vi "启动整机测试 (子VI).vi"() -> (0 "error out":T1={"status"=FALSE, "代码"=4, "source"=""} caption="错误输出" {"代码" items=["执行成功"=1, "执行失败，但不知道原因"=2, "命令请求条件错误"=3, "通讯超时"=4, "系统繁忙不能执行"=5, "系统故障"=6, "没有数据"=100]})   [LabVIEW 2016, in "MB SLAVE.lvlib"]
uses:
  MB SLAVE.lvlib
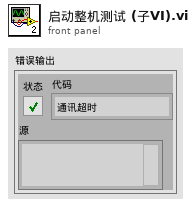
[diagram p1: front panel]
types:
  T1 = cluster{"status":bool, "代码":u16, "source":string}
  T2 = typedef "系统交互.ctl" = cluster{"运行模式":enum16{"维护模式", "常规模式", "应急模式", "质控模式"}, "运行间隔":i16, "流程运行中":bool, "自动运行启动参数":bool[], "SYSTEM Interface.总磷总氮类型":enum16{"单模块", "总磷总氮二合一模块", "氨氮总磷二合一模块"}, "多参数运行间隔":i16}
  T3 = cluster{"参数启用":cluster{"氨氮":bool, "总磷":bool, "总氮":bool, "多参数":bool, "CODMn":bool, "CODcr":bool, "超标留样":bool}}
  T4 = cluster{"自动运行启动参数[0]":bool, "自动运行启动参数[1]":bool, "自动运行启动参数[2]":bool, "自动运行启动参数[3]":bool, "自动运行启动参数[4]":bool, "自动运行启动参数[5]":bool, "自动运行启动参数[6]":bool}
  T5 = cluster{"自动运行启动参数":cluster{"自动运行启动参数[0]":bool, "自动运行启动参数[1]":bool, "自动运行启动参数[2]":bool, "自动运行启动参数[3]":bool, "自动运行启动参数[4]":bool, "自动运行启动参数[5]":bool, "自动运行启动参数[6]":bool}}
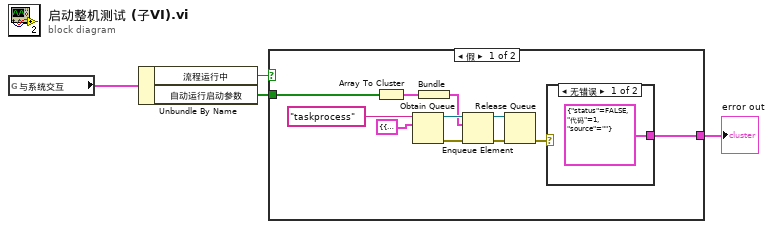
[diagram p0: block diagram]
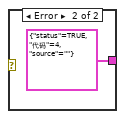
[diagram p2: hidden frame]
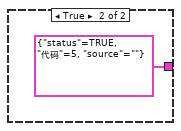
[diagram p3: hidden frame]
diagram:
  n1 = global read "modbus slave全局.vi" "与系统交互"() -> (w3:T2)
  n2 = Unbundle By Name(w3) -> ("流程运行中"=w2:bool, "自动运行启动参数"=w1:bool[])
  n3 = case shown="假" w2 {
    tunnel: [w15 T1 {"status"=TRUE, "代码"=5, "source"=""} ("error out")] -> w4
    tunnel: w1 -> [w6 _]
    frame False {
      n4 = Array To Cluster(array=w6) -> (cluster=w5:T4)
      n5 = Obtain Queue(name (unnamed)="taskprocess" ("名称（未命名）"), element data type=T3 {"参数启用"={"氨氮"=FALSE, "总磷"=FALSE, "总氮"=FALSE, "多参数"=FALSE, "CODMn"=FALSE, "CODcr"=FALSE, "超标留样"=FALSE}} ("参数")) -> (queue out=w12:refnum<queue>, error out=w11:errorcluster)  [unwired: 3 in, 1 out]
      n6 = Bundle("自动运行启动参数"=w5) -> (w10:T5)  [unwired: 1 in]
      n7 = Enqueue Element(queue=w12, element=w10, error in (no error)=w11) -> (queue out=w8:refnum<queue>, error out=w9:errorcluster)  [unwired: 1 in, 1 out]
      n8 = Release Queue(queue=w8, error in (no error)=w9) -> (error out=w7:errorcluster)  [unwired: 1 in, 2 out]
      n9 = case shown="无错误" w7 {
        tunnel: [T1 {"status"=FALSE, "代码"=1, "source"=""} ("error out") T1 {"status"=TRUE, "代码"=4, "source"=""} ("error out")] -> w15
        frame No Error {
        }
        frame Error {
        }
      }
    }
    frame True {
    }
  }
  "error out" <- w4
